vi "GetCountOfTransactionsInOutNak.vi"(2 "Colors":u32[](array[colorbox])=[11796480, 37103, 40712, 16770816, 11796658, 4210752]) -> (1 "Percent %":dbl[](array[numeric]) format="%.2f", 3 "Pie Chart Transactions: In - Out- Nak":picture)   [LabVIEW 2014]
uses:
  USBAnalyzerEllisysDll/Debug/USBAnalyzerEllisysDll.dll
panel:
  out "return type":i32
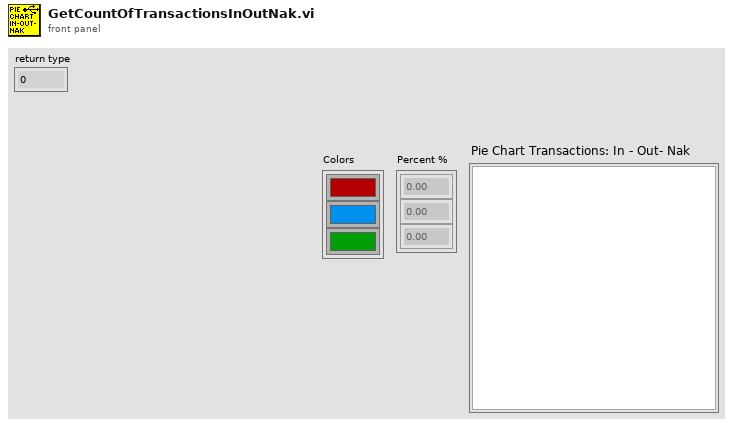
[diagram p1: front panel]
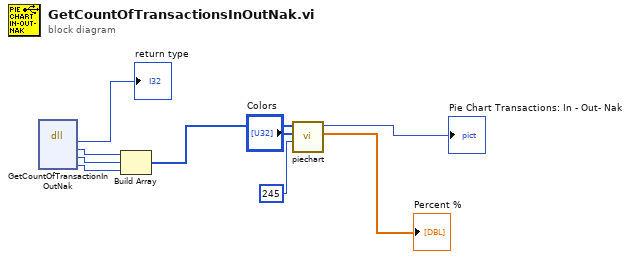
[diagram p0: block diagram]
diagram:
  n1 = dll-call lib="PTH2labs CUsersMichał\tDocumentsEllisysAnalyzerUSBAnalyzerEllisysDllDebugUSBAnalyzerEllisysDll.dll" fn="GetCountOfTransactionInOutNak"() -> ("return type"=→"return type":i32, "in"=w7:u64, "out"=w6:u64, "nak"=w5:u64)  [unwired: 6 in, 2 out]
  n2 = Build Array(w7, w6, w5) -> (w4:u64[])
  n3 = call "piechart.vi"("Pie Chart Size"=i16 245, "Colors"="Colors", "Values"=w4) -> ("Percent %"=→"Percent %":dbl[], "Pie Chart"=→"Pie Chart Transactions: In - Out- Nak":picture)  [unwired: 5 in]
